vi "test_SessionInitializeErrors_CallInitializeSessionsForRemoteSession_InitializeRetriesAndSucceeds.vi"() -> ()   [LabVIEW 2020, in "MeasurementServerTests.lvlib"]
uses:
  MeasurementServerTests.lvlib
  d8d5ad7a-7c66-4327-8078-b5d2e2b8507a.vi
  Runtime/MeasurementLink niDCPower/Create Sessions - NSess.vi
  Runtime/MeasurementLink niDCPower/MeasurementLink niDCPower.lvlib
  Runtime/MeasurementLink Session Management/Session Reservation/Session Reservation.lvclass
panel:
  in  "error in":errorcluster
  out "result":string
  out "pass":bool
  out "error out":errorcluster
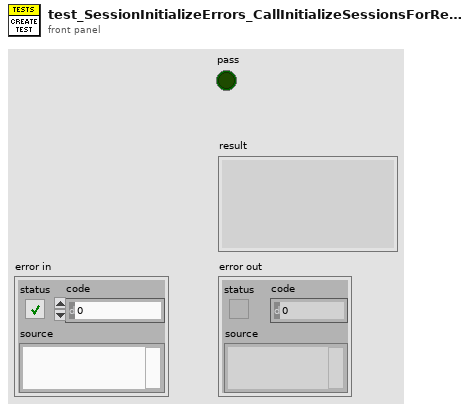
[diagram p1: front panel]
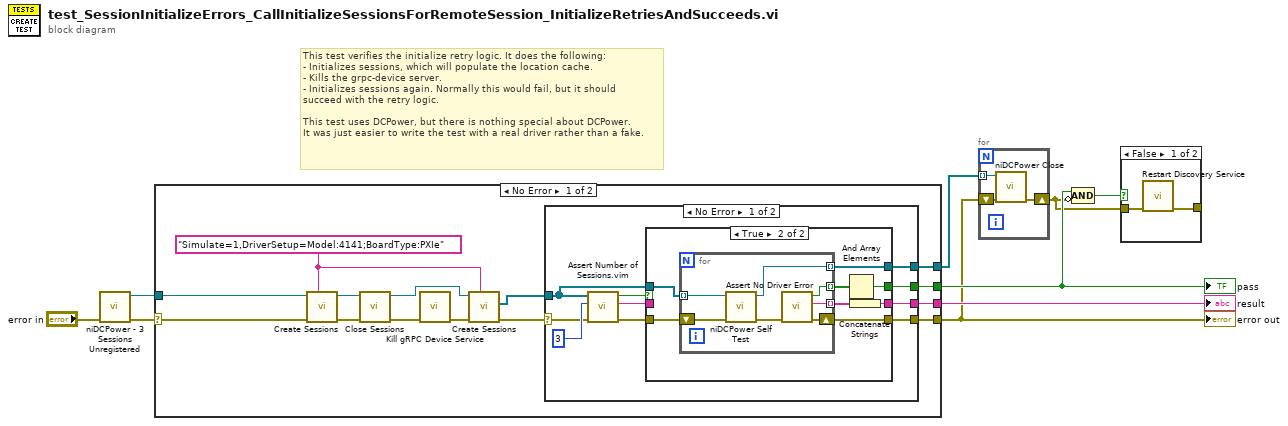
[diagram p0: block diagram]
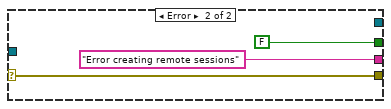
[diagram p4: hidden frame]
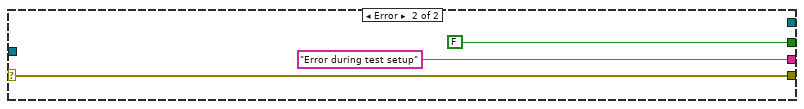
[diagram p5: hidden frame]
diagram:
  # "This test verifies the initialize retry logic. It does the following:\n- Initializes sessions, which will populate the location cache.\n- Kills the grpc-device server.\n- Initializes sessions again. Normally this would fail, but it should\nsucceed with the retry logic.\n\nThis test uses DCPower, but there is nothing special about DCPower.\nIt was just easier to write the test with a real driver rather than a fake."
  n1 = call "niDCPower - 3 Sessions Unregistered.vi"("error in (no error)"="error in") -> ("error out"=w6:errorcluster, "Session Reservation out"=w5:refnum<class "Session Reservation.lvclass">)  [unwired: 9 in]
  n2 = case shown="No Error" w6 {
    selector: w6 -> [w18 w56]
    tunnel: [w22 w56] -> w2
    tunnel: [w23 FALSE] -> w3
    tunnel: [w21 "Error during test setup" ("f")] -> w9
    tunnel: [w20 _] -> w8
    tunnel: w5 -> [w19 _]
    frame No Error {
      w14 = "Simulate=1,DriverSetup=Model:4141;BoardType:PXIe" ("option string")
      n3 = call-poly "Create Sessions.vi"("option string"=w14, "error in"=w18, "session reservation in"=w19) -> ("error out"=w16:errorcluster, "session reservation out"=w15:refnum<class "Session Reservation.lvclass">)  [unwired: 5 in, 2 out]
      n4 = call "Close Sessions.vi"("error in"=w16, "session reservation in"=w15) -> ("error out"=w13:errorcluster, "session reservation out"=w12:refnum<class "Session Reservation.lvclass">)  [unwired: 8 in]
      n5 = call "Kill gRPC Device Service.vi"("error in"=w13) -> ("error out"=w17:errorcluster)  [unwired: 10 in]
      n6 = call-poly "Create Sessions.vi"("option string"=w14, "error in"=w17, "session reservation in"=w12) -> ("error out"=w11:errorcluster, "sessions"=w10:refnum<k15>[])  [unwired: 5 in, 2 out]
      n7 = case shown="No Error" w11 {
        selector: w11 -> [w27 w54]
        tunnel: [w28 FALSE] -> w23
        tunnel: [w32 w54] -> w22
        tunnel: [w33 "Error creating remote sessions"] -> w21
        tunnel: [w31 _] -> w20
        tunnel: w10 -> [w30 _]
        frame No Error {
          n8 = call "Assert Number of Sessions.vim"("error in"=w27, "expected number of sessions"=3 ("y"), "sessions"=w30) -> ("error out"=w26:errorcluster, "result"=w24:string, "pass"=w25:bool)  [unwired: 6 in]
          n9 = case shown="True" w25 {
            selector: w25 -> [w37 _]
            tunnel: [w36 w38] -> w33
            tunnel: [w35 w43] -> w32
            tunnel: [w34 w42] -> w31
            tunnel: w30 -> [w34 w41]
            tunnel: [w37 w39] -> w28
            tunnel: w26 -> [w35 w40]
            tunnel: w24 -> [w36 _]
            frame False {
            }
            frame True {
              n10 = for {
                tunnel: [w52] -> w45 mode=indexing
                tunnel: [w51] -> w44 mode=indexing
                tunnel: [w49] -> w42 mode=indexing
                tunnel: w41 -> [w47] mode=indexing
                shift-right: [w50] -> w43
                shift-left: w40 -> [w46]
                n11 = call <instrlib>:"niDCPower Self Test.vi"("error in (no error)"=w46, "instrument handle"=w47) -> ("error out"=w48:errorcluster, "instrument handle out"=w49:refnum<k15>)  [unwired: 6 in, 2 out]
                n12 = call "Assert No Driver Error.vi"("error in"=w48) -> ("error out"=w50:errorcluster, "result"=w51:string, "pass?"=w52:bool)  [unwired: 8 in]
              }
              n13 = And Array Elements(Boolean array=w45) -> (logical AND=w39:bool)
              n14 = Concatenate Strings(w44) -> (w38:string)
            }
          }
        }
        frame Error {
        }
      }
    }
    frame Error {
    }
  }
  "error out" <- w2
  "pass" <- w3
  "result" <- w9
  n15 = for {
    tunnel: w8 -> [w61] mode=indexing
    shift-right: [w60] -> w1
    shift-left: w2 -> [w59]
    n16 = call <instrlib>:"niDCPower Close.vi"("error in (no error)"=w59, "instrument handle"=w61) -> ("error out"=w60:errorcluster)  [unwired: 9 in]
  }
  n17 = Compound Arithmetic op=AND(w3, invert w1) -> (w4:bool)
  n18 = case shown="False" w4 {
    tunnel: [w63 _] -> _
    tunnel: w1 -> [w62 _]
    frame False {
      n19 = call "Restart Discovery Service.vi"("error in"=w62) -> ("error out"=w63:errorcluster)  [unwired: 10 in]
    }
    frame True {
    }
  }
